vi "to string.vi"(8 "error in":errorcluster, 11 "user tag bus module configuration In":refnum<class "user tag bus module configuration.lvclass">) -> (0 "error out":errorcluster, 1 "data":string, 2 "version":string, 3 "user tag bus module configuration Out":refnum<class "user tag bus module configuration.lvclass">)   [LabVIEW 2013, in "user tag bus module configuration.lvclass"]
doc: "Provides an interface for saving a module configuration to a file or other serialized data source. It is recommended that all children of this class store data in two sets--data required for its own initialization, and any data required for parent initialization--and that each implementation uses the <b>Call Parent Method</b> primitive to serialize parent information."
uses:
  user tag bus module configuration.lvclass
  <vilib>/NI/Tag Bus Module Framework/module configuration/TBM module configuration.lvclass
  <vilib>/NI/Configuration Framework/serializable configuration/NISE_CEF_serializable configuration.lvclass
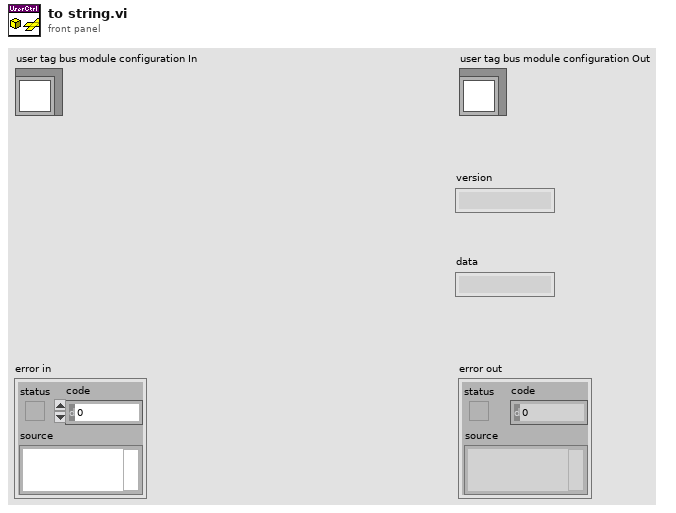
[diagram p1: front panel]
types:
  T1 = typedef "user tag bus module configuration.lvclass/state module configuration.ctl" = cluster{"fixed input":refnum<class "TBM channel.lvclass">, "fixed output":refnum<class "TBM channel.lvclass">, "initial state":u8}
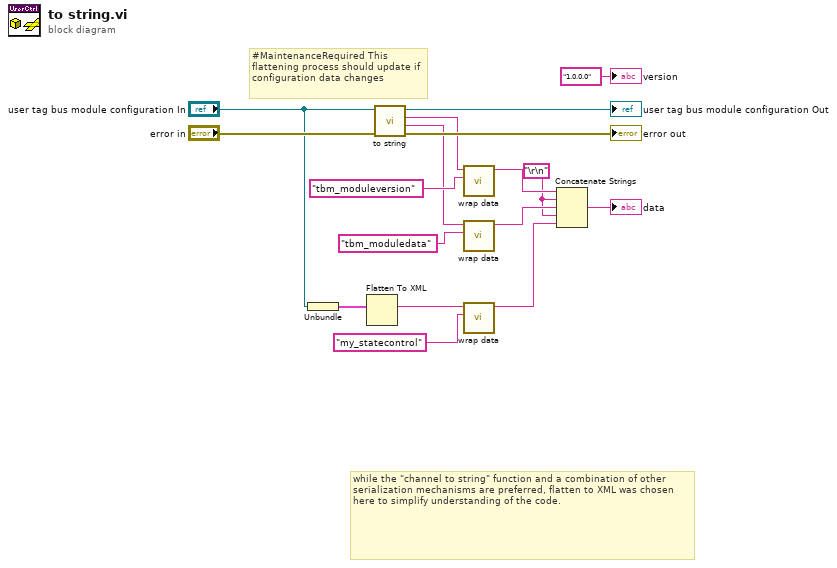
[diagram p0: block diagram]
diagram:
  w2 = "\r\n"
  # "while the \"channel to string\" function and a combination of other serialization mechanisms are preferred, flatten to XML was chosen here to simplify understanding of the code."
  # "#MaintenanceRequired This flattening process should update if configuration data changes"
  n1 = Unbundle("user tag bus module configuration In") -> (w3:T1)
  n2 = Flatten To XML(anything=w3) -> (xml string=w6:string)
  n3 = call-parent "to string.vi"("error in"="error in", "module configuration in"="user tag bus module configuration In") -> ("error out"=→"error out":errorcluster, "data"=w9:string, "version"=w10:string, "module configuration out"=→"user tag bus module configuration Out":refnum<class "user tag bus module configuration.lvclass">)  [unwired: 6 in]
  n4 = call <vilib>:"wrap data.vi"("identifier"="tbm_moduleversion" ("additional identifier"), "data to wrap"=w10) -> ("wrapped data"=w12:string)  [unwired: 9 in]
  n5 = call <vilib>:"wrap data.vi"("identifier"="tbm_moduledata" ("additional identifier"), "data to wrap"=w9) -> ("wrapped data"=w11:string)  [unwired: 9 in]
  n6 = call <vilib>:"wrap data.vi"("identifier"="my_statecontrol" ("additional identifier"), "data to wrap"=w6) -> ("wrapped data"=w5:string)  [unwired: 9 in]
  n7 = Concatenate Strings(w12, w2, w11, w2, w5) -> (→"data":string)
  "version" <- "1.0.0.0" ("version")
